vi "ChangeDispensing.vi"() -> ()   [LabVIEW 2016]
uses:
  Other Models/EFD Ultimus V/EFD Ultimus V.lvlib
panel:
  in  "VISA resource name":refnum<visa-resource-name>="COM5"
  in  "Serial Configuration":T1={"Baud Rate "=115200, "Parity "=0, "Data Bits "=8, "Stop Bits"=10} {"Stop Bits" items=["1.0"=10, "1.5"=15, "2.0"=20]; "Data Bits" items=["7"=7, "8"=8]; "Parity" items=["None", "Odd", "Even"]; "Baud Rate" items=["9600"=9600, "19200"=19200, "38400"=38400, "115200"=115200]}
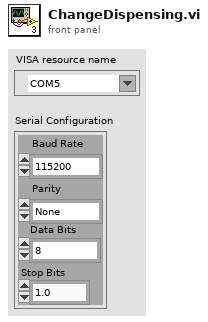
[diagram p1: front panel]
types:
  T1 = cluster{"Baud Rate ":u32, "Parity ":u16, "Data Bits ":u16, "Stop Bits":u16}
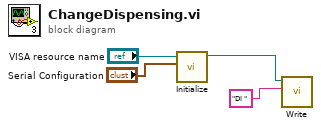
[diagram p0: block diagram]
diagram:
  n1 = call "Initialize.vi"("Serial Configuration"="Serial Configuration", "VISA resource name"="VISA resource name") -> ("VISA resource name out"=w2:refnum<visa-resource-name>)  [unwired: 8 in, 1 out]
  n2 = call "Write.vi"("Command To Write"="DI ", "VISA resource name"=w2) -> ()  [unwired: 8 in, 2 out]
